vi "Set_Parameter_Instrument (Json).vi"(8 "error in (no error)":errorcluster caption="entrée d'erreur (pas d'erreur)", 10 "Parameter (Json)":string, 11 "Flash_Jlink en entrée":refnum<class "Flash_Jlink.lvclass">) -> (0 "error out":errorcluster caption="sortie d'erreur", 3 "Flash_Jlink en sortie":refnum<class "Flash_Jlink.lvclass">)   [LabVIEW 2020, in "Library Test.lvlib" / "Flash_Jlink.lvclass"]
uses:
  Flash_Jlink.lvclass
  C:/Users/ngarcin/OneDrive - Altyor/Standard TB/Class/Test/Test (Default)/Test (Default).lvclass
  Commun VI/TypeDef/Commande Test/Commande Parameter Flash_Jlink.ctl
  Flash_Jlink.lvclass/Flash_Jlink.ctl
  JSON API/JSON Value/Set from JSON string.vi
  Test_Without_Instr/Test_Without_Inst.lvclass
  JSON API/JSON Value/JSON Value.lvclass
  Commun VI/Library Commun.lvlib
  JSON API/Variant JSON/Variant JSON.lvlib
  JSON API/Get Polymorphic/JSON GetSet.lvlib
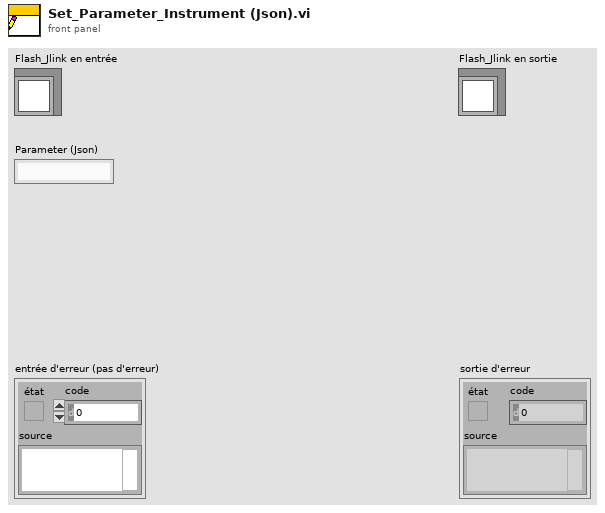
[diagram p1: front panel]
types:
  T1 = typedef "Library Commun.lvlib/Commande Parameter Flash_Jlink.ctl" = cluster{"Path FW":path, "Working Directory":path, "Device":string, "Frequency":string, "Connection_Type":string}
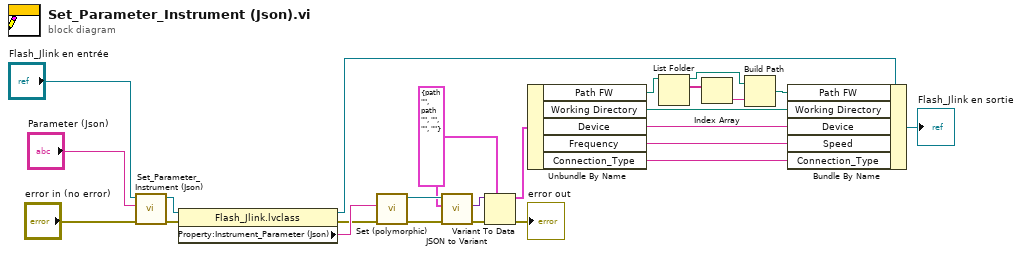
[diagram p0: block diagram]
diagram:
  w15 = T1 {"Path FW"=path "", "Working Directory"=path "", "Device"="", "Frequency"="", "Connection_Type"=""}
  n1 = call-parent "Set_Parameter_Instrument (Json).vi"("error in (no error)"="error in (no error)", "Parameter (Json)"="Parameter (Json)", "Test (Default) en entrée"="Flash_Jlink en entrée") -> ("error out"=w14:errorcluster, "Test (Default) en sortie"=w17:refnum<class "Flash_Jlink.lvclass">)  [unwired: 7 in]
  n2 = property class="Flash_Jlink.lvclass"(reference=w17, error in=w14) -> (reference out=w13:refnum<class "Flash_Jlink.lvclass">, error out=w11:errorcluster, "Property:Instrument_Parameter (Json)"=w16:string)
  n3 = call-poly "Set (polymorphic).vi"("error in (no error)"=w11, "JSON stream"=w16) -> ("error out"=w19:errorcluster, "JSON Value out"=w21:refnum<class "JSON Value.lvclass">)  [unwired: 7 in, 1 out]
  n4 = call "JSON to Variant.vi"("error in (no error)"=w19, "Variant (Data Type)"=w15, "JSON Value"=w21) -> ("error out"=w20:errorcluster, "Variant out"=w18:variant)  [unwired: 7 in]
  n5 = Variant To Data(error in=w20, type=w15, Variant=w18) -> (data=w12:T1, error out=→"error out":errorcluster)
  n6 = Unbundle By Name(w12) -> ("Path FW"=w1:path, "Working Directory"=w9:path, "Device"=w8:string, "Frequency"=w7:string, "Connection_Type"=w6:string)
  n7 = List Folder(path=w1) -> (path out=w4:path, filenames=w5:string[])  [unwired: 3 in, 2 out]
  n8 = Index Array(array=w5) -> (element=w2:string)  [unwired: 1 in]
  n9 = Build Path(base path=w4, name or relative path=w2) -> (appended path=w3:path)
  n10 = Bundle By Name(cluster=w13, "Path FW"=w3, "Working Directory"=w9, "Device"=w8, "Speed"=w7, "Connection_Type"=w6) -> (→"Flash_Jlink en sortie":refnum<class "Flash_Jlink.lvclass">)
